vi "CRIS responder.vi"() -> ()   [LabVIEW 2013]
panel:
  out "waveSet":dbl
  out "isNew":bool
  out "waveReadback":dbl
  in  "stop":bool
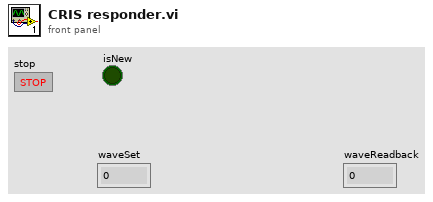
[diagram p1: front panel]
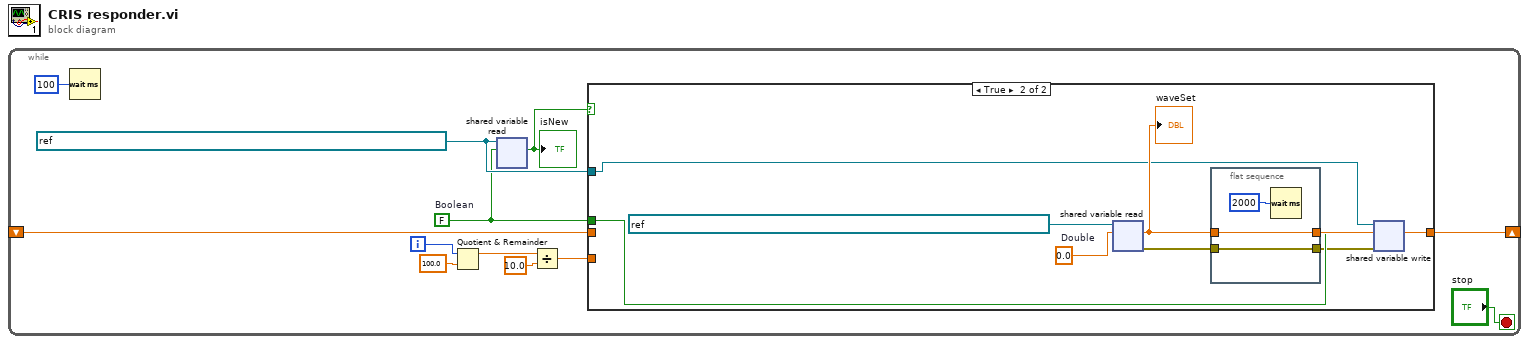
[diagram p0: block diagram]
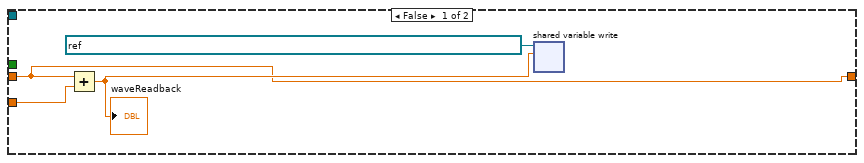
[diagram p2: hidden frame]
diagram:
  n1 = while {
    shift-right: [w5] -> _
    shift-left: _ -> [w4]
    i -> [w10]
    stop <- "stop" stop-if-true
    w2 = FALSE  # Boolean
    w3 = refnum<k21> "ni.var.psp://localhost/Narrow Band TiSa Scanner Shared Variables/isNew" ("shared variable refnum in")
    n2 = Wait (ms)(milliseconds to wait=u32 100) -> ()  [unwired: 1 out]
    n3 = Quotient & Remainder(x=w10, y=100.0) -> (x-y*floor(x/y)=w7:dbl)  [unwired: 1 out]
    n4 = shared-variable-read(w3, w2) -> (w12:bool)  [unwired: 1 in, 3 out]
    "isNew" <- w12
    n5 = Divide(x=w7, y=10.0) -> (x/y=w6:dbl)
    n6 = case shown="True" w12 {
      tunnel: [w13 w21] -> w5
      tunnel: w6 -> [w16 _]
      tunnel: w4 -> [w13 _]
      tunnel: w3 -> [_ w20]
      tunnel: w2 -> [_ w19]
      frame False {
        n7 = Add(x=w13, y=w16) -> (x+y=w14:dbl)
        "waveReadback" <- w14
        n8 = shared-variable-write(refnum<k21> "ni.var.psp://localhost/Narrow Band TiSa Scanner Shared Variables/waveReadback" ("shared variable refnum in"), w14) -> ()  [unwired: 1 in, 2 out]
      }
      frame True {
        w23 = 0.0  # Double
        n9 = shared-variable-read(refnum<k21> "ni.var.psp://localhost/Narrow Band TiSa Scanner Shared Variables/waveSet" ("shared variable refnum in"), w23) -> (w17:errorcluster, w22:dbl)  [unwired: 1 in, 2 out]
        "waveSet" <- w22
        n10 = flat-sequence {
          tunnel: [w26] -> w21
          tunnel: w22 -> [w26]
          tunnel: [w25] -> w18
          tunnel: w17 -> [w25]
          frame #0 {
            n11 = Wait (ms)(milliseconds to wait=u32 2000) -> ()  [unwired: 1 out]
          }
        }
        n12 = shared-variable-write(w20, w18, w19) -> ()  [unwired: 2 out]
      }
    }
  }
